vi "ReturnMovePattern.vi"(8 "error in (no error)":errorcluster, 11 "object in":refnum<class "Piece.lvclass">) -> (0 "error out":errorcluster, 3 "object out":refnum<class "Piece.lvclass">)   [LabVIEW 2020, in "Piece.lvclass"]
doc: "returns the moving pattern of the piece"
uses:
  Piece.lvclass
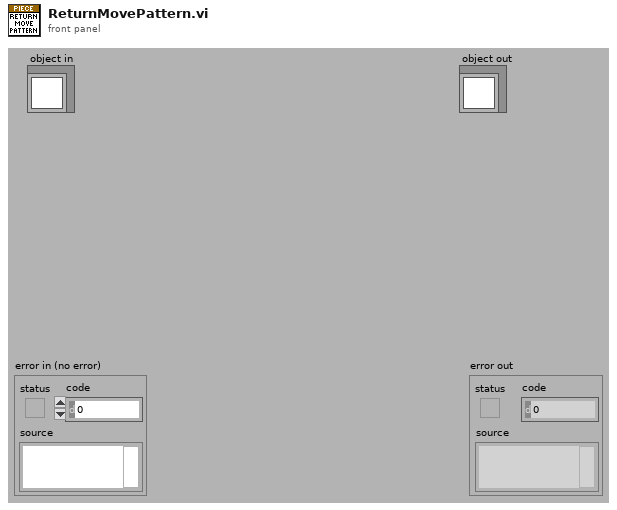
[diagram p1: front panel]
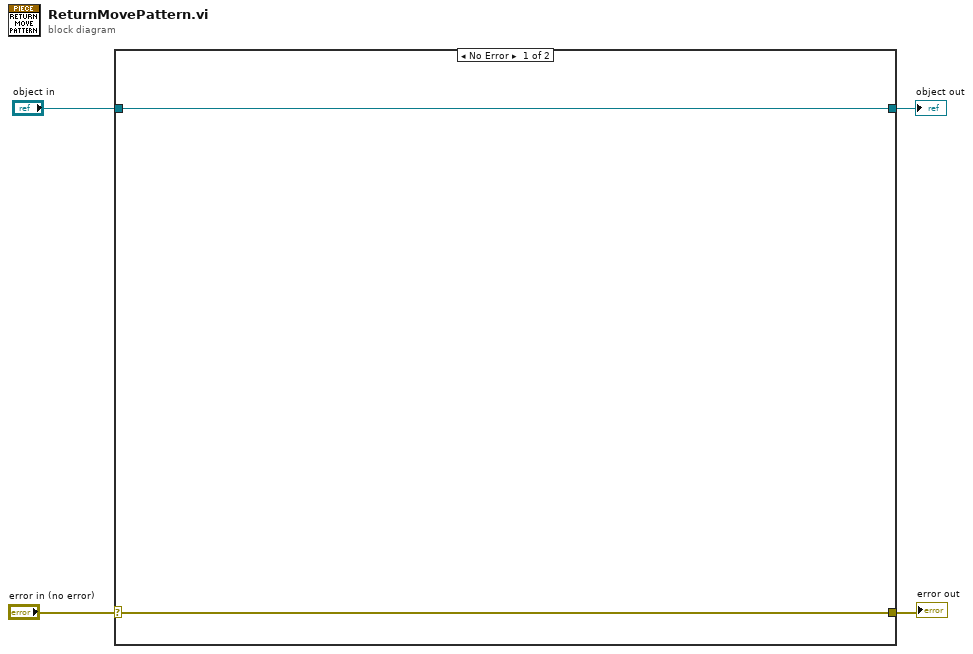
[diagram p0: block diagram]
diagram:
  n1 = case shown="No Error" "error in (no error)" {
    selector: "error in (no error)" -> [w5 w8]
    tunnel: [w5 w8] -> w3
    tunnel: [w6 w7] -> w1
    tunnel: "object in" -> [w6 w7]
    frame No Error {
    }
    frame Error {
    }
  }
  "error out" <- w3
  "object out" <- w1
